vi "LiveSignal.vi"() -> ()   [LabVIEW 2022 SP3]
uses:
  <extravilib>/ChannelInstances/Tag-a[.](wfm(dbl)).lvlib
  ViolinSubs/Mic/Mic_Global.vi
  <extravilib>/ChannelInstances/Lossy Stream-a[.](wfm(dbl)).lvlib
  <vilib>/Analysis/NI_AALPro.lvlib
  ViolinSubs/PreferencesControl.ctl
panel:
  in  "Update Template":bool
  in  "max_scale":bool
  in  "last scale":bool
  in  "Load a Template":bool
  in  "autoscale":bool
  in  "Save as a Template":bool
  in  "device:":u16(ring) items=["BuerginBase Microphone", "485B39 200083408035100798118210422", "MacBook Pro Microphone", "Camo Microphone", "KM Audio Device", "Microsoft Teams Audio", "ZoomAudioDevice"]
  out "data":waveform(dbl)[](array[waveform])
  in  "Tab Control":T1(tab)
  in  "Magnitude Averages":u8(slide)=25 scale=1.0..50.0
  out "Hammer":waveform(dbl)(graph)
  out "Microphone":waveform(dbl)(graph)
  out "Mic Power Spectrum":waveform(dbl)(graph)
  out "Cal Hammer":waveform(dbl)[](graph)
  out "cal Mic":waveform(dbl)[](graph)
  out "Power Spectrum 2":waveform(dbl)(graph)
  in  "In->Out":bool
  in  "Out->In":bool
  out "Trig Mic":waveform(dbl)[](graph)
  out "Trig Hammer":waveform(dbl)[](graph)
  out "Triggered Spectrum":waveform(dbl)(graph)
  out "Real/Imag":cluster{dbl, "df":dbl, dbl[]}[](graph)
  out "Average FRF":cluster{dbl, "df":dbl, dbl[]}(graph)
  in  "Offset (msec)":dbl(slide) scale=0.0..10.0
  in  "Settings":T2={"Name of test"="", "Date"=timestamp(3691169924 s since 1904-01-01), "Location"="", "Template"="", "Soundcard"="485B39 200083408035100798118210422", "resolution"=32, "Sampling rate"=48000, "Ch1 Gain "=0.0, "Ch2 Gain"=0.0, "Sample time (s)"=0.3, "Pre-trigger (s)"=0.01, "Hammer Threshold"=0.01, "Positions"=12, "Taps/Position"=5, "Set Names"="", "Freq resolution"=1.0, "Hammer cutoff"=1.0, "Mic cutoff"=1.0, "Double bounce "=0.1, "Hammer Cal"=1000.0, "dB Offset"=0.0, "Accel Cal"=1000.0, "Vibrometer Cal"=1000.0, "Mic Cal"=1000.0, "Output"=2, "Voltage Cal"=1.0, "Vibrometer Port"="ASRL27::INSTR", "Range"=50, "High Pass"=2, "Bandwidth"=25, "X Range"=[], "Y Range"=[], "dB Spread"=40.0, "Trigger"=0, "Ch_1"=1, "Ch_2"=2, "flip?"=FALSE, "60Hz"=FALSE, "Time offset"=0.0, "Piezo Cal"=1.0, "Default Notes"="", "Tom"=FALSE} {"Ch_2" min=1 step=1; "Ch_1" min=1 max=100 step=1; "Trigger" items=["Hammer (force)", "Self-tap", "Spacebar"]; "Bandwidth" items=["1 kHz"=1, "5 kHz"=5, "10 kHz"=10, "25 kHz"=25, "50 kHz"=50, "100 kHz"=100]; "High Pass" items=["Off", "13 Hz", "104 Hz"]; "Range" items=["10 mm/s"=1, "20 mm/s"=2, "50 mm/s"=5, "100 mm/s"=10, "200 mm/s"=20, "500 mm/s"=50, "1 m/s"=100, "2 m/s"=200]; "Output" items=["Accelerometer", "Speed (from acceleration)", "Microphone", "Vibrometer", "Piezo"]; "Voltage Cal" format="%#_13g"; "Ch2 Gain" format="%#_13g"; "Ch1 Gain" format="%#_13g"; "Double bounce" min=0.0; "Mic cutoff" min=0.0 format="%#_4g"; "Hammer cutoff" min=0.0 format="%#_4g"; "Freq resolution" min=0.0; "Pre-trigger (s)" format="%#_13g"; "Date" format="%<%H:%M\n%d/%m/%y>T"; "resolution" items=["16 bit"=16, "24 bit"=24, "32 bit"=32]; "Sampling rate" items=["22050 samp/s"=22050, "44100 samp/s"=44100, "48000 samp/s"=48000]}
  # "For Mac mic - start running and then have both channels on 1"
  # "Raw values from the Soundcard"
  # "Calibrated Values"
  # "All values are calibrated, arrows sync x axes"
  # "Hz"
  # "dB"
  # "dB"
  # "sec"
  # "sec"
  # "mV/Pa"
  # "mV/m/s2"
  # "mV/mm/s"
  # "V/N"
  # "sec"
  # "sec"
  # "mV/N"
  # "%"
  # "%"
  # "sec"
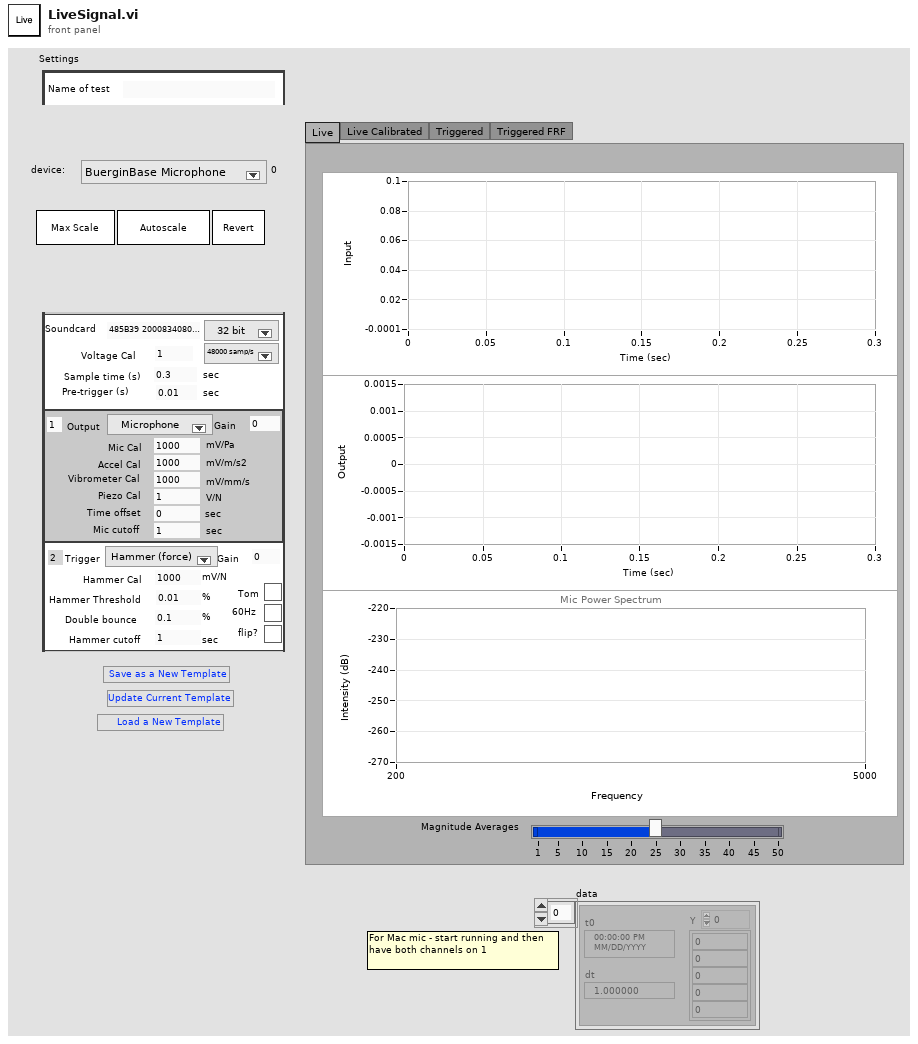
[diagram p1: front panel]
types:
  T1 = enum32{"Live", "Live Calibrated", "Triggered", "Triggered FRF"}
  T2 = typedef "PreferencesControl.ctl" = cluster{"Name of test":string, "Date":timestamp, "Location":string, "Template":string, "Soundcard":string, "resolution":u16, "Sampling rate":u16, "Ch1 Gain ":dbl, "Ch2 Gain":dbl, "Sample time (s)":dbl, "Pre-trigger (s)":dbl, "Hammer Threshold":dbl, "Positions":i16, "Taps/Position":i16, "Set Names":string, "Freq resolution":dbl, "Hammer cutoff":dbl, "Mic cutoff":dbl, "Double bounce ":dbl, "Hammer Cal":dbl, "dB Offset":dbl, "Accel Cal":dbl, "Vibrometer Cal":dbl, "Mic Cal":dbl, "Output":u16, "Voltage Cal":dbl, "Vibrometer Port":refnum<visa-resource-name>, "Range":u16, "High Pass":u16, "Bandwidth":u16, "X Range":cluster{"Minimum":dbl, "Maximum":dbl, "Increment":dbl, "Minor Increment":dbl, "Start":dbl}[], "Y Range":cluster{"Minimum":dbl, "Maximum":dbl, "Increment":dbl, "Minor Increment":dbl, "Start":dbl}[], "dB Spread":dbl, "Trigger":u16, "Ch_1":u8, "Ch_2":u8, "flip?":bool, "60Hz":bool, "Time offset":dbl, "Piezo Cal":dbl, "Default Notes":string, "Tom":bool}
  T3 = typedef "Tag-a[.](wfm(dbl)).lvlib/))Channel.ctl" = refnum<queue>
  T4 = typedef "Lossy Stream-a[.](wfm(dbl)).lvlib/)Channel.ctl" = refnum<queue>
  T5 = enum8{"Enabled", "Disabled", "Disabled and Grayed Out"}
  T6 = enum16{"Read", "Write", "Init", "remember", "retrieve"}
  T7 = typedef "LVRangeTypeDef.ctl" = cluster{"Minimum":dbl, "Maximum":dbl, "Increment":dbl, "Minor Increment":dbl, "Start":dbl}
  T8 = enum16{"Initialize", "Free run", "One Shot - waiting", "One Shot - triggered", "Wait", "Close"}
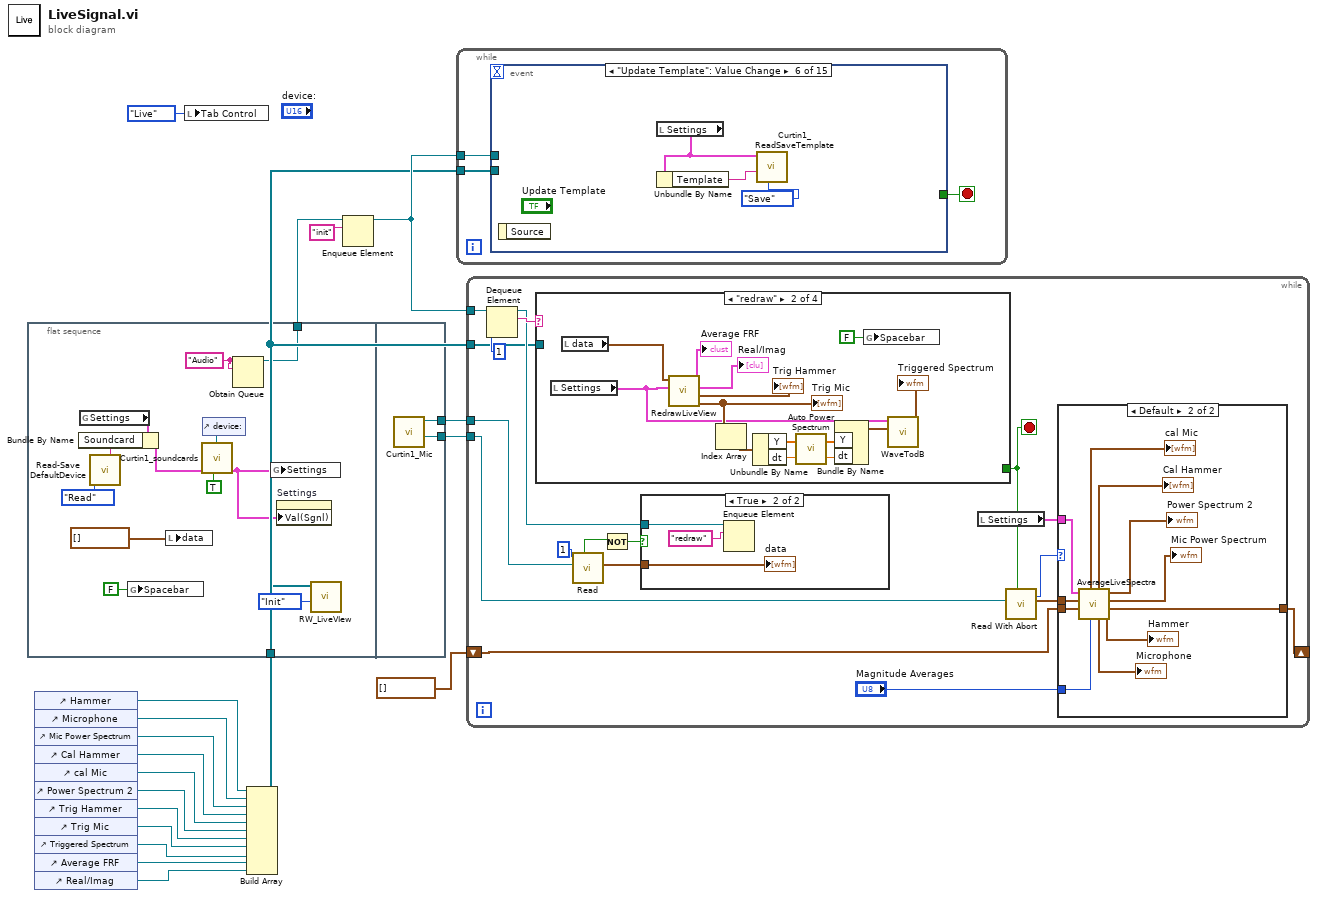
[diagram p0: block diagram]
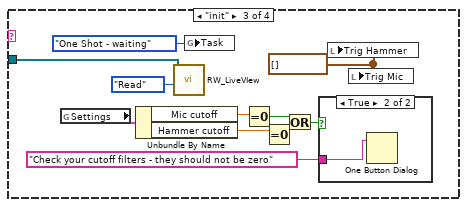
[diagram p5: hidden frame]
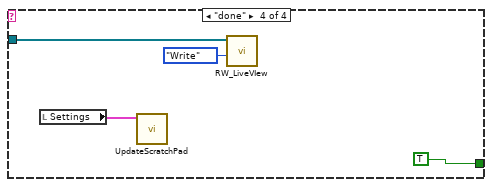
[diagram p7: hidden frame]
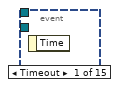
[diagram p8: hidden frame]
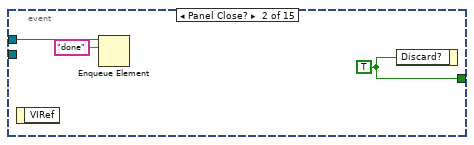
[diagram p9: hidden frame]
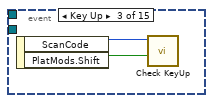
[diagram p10: hidden frame]
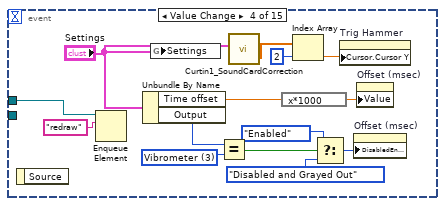
[diagram p11: hidden frame]
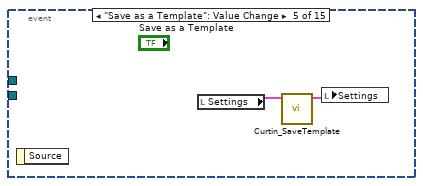
[diagram p12: hidden frame]
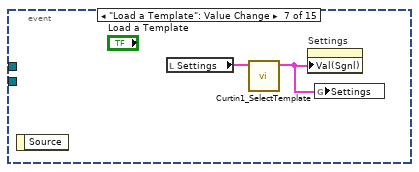
[diagram p13: hidden frame]
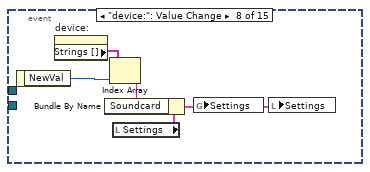
[diagram p14: hidden frame]
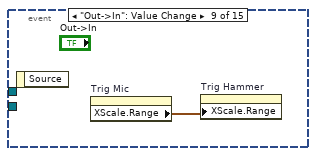
[diagram p15: hidden frame]
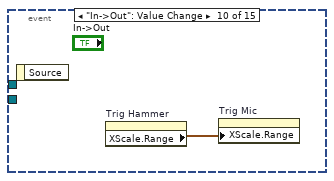
[diagram p16: hidden frame]
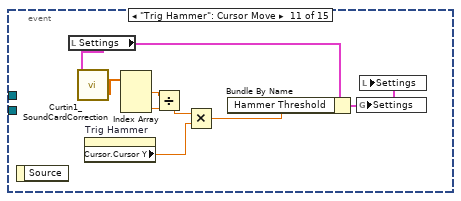
[diagram p17: hidden frame]
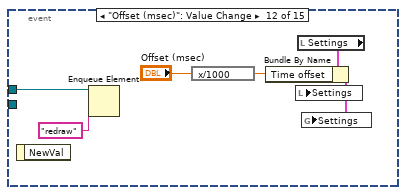
[diagram p18: hidden frame]
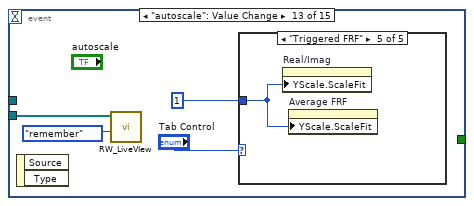
[diagram p19: hidden frame]
diagram:
  n1 = flat-sequence {
    tunnel: [w26] -> w15
    tunnel: w1 -> [w22]
    tunnel: [w34] -> w19
    tunnel: [w33] -> w18
    frame #0 {
      w27 = "Audio" ("name (unnamed)")
      n2 = global read "Mic_Global.vi" "Settings"() -> (w30:T2)
      n3 = call "Read-Save DefaultDevice.vi"("Task"=enum16{"Save", "Read"}."Read") -> ("Soundcard Out"=w29:string)  [unwired: 9 in, 1 out]
      n4 = Bundle By Name(cluster=w30, "Soundcard"=w29) -> (w25:T2)
      n5 = global write "Mic_Global.vi" "Spacebar"(FALSE ("Spacebar")) -> ()
      n6 = local write "data"(waveform(dbl)[] [] ("data")) -> ()
      n7 = control-ref of="device:"() -> (w32:refnum<vi>)
      n8 = call "Curtin1_soundcards.vi"("hush?"=TRUE, "Settings In"=w25, "device:"=w32) -> ("Settings Out"=w24:T2)  [unwired: 7 in, 1 out]
      n9 = Obtain Queue(name (unnamed)=w27, element data type=w27) -> (queue out=w26:refnum<queue>)  [unwired: 3 in, 2 out]
      n10 = global write "Mic_Global.vi" "Settings"(w24) -> ()
      n11 = property on="Settings" class="Clust (strict)"("Val(Sgnl)"=w24) -> ()  [unwired: 2 in, 2 out]
      n12 = call "RW_LiveVIew.vi"("Task"=enum16{"Read", "Write", "Init"}."Init", "Plots"=w22) -> ()  [unwired: 10 in]
    }
    frame #1 {
      n13 = call "Curtin1_Mic.vi"() -> ("latest data"=w33:T3, "Tap"=w34:T4)  [unwired: 10 in]
    }
  }
  n14 = control-ref of="Hammer"() -> (w13:refnum<vi>)
  n15 = control-ref of="Microphone"() -> (w12:refnum<vi>)
  n16 = control-ref of="Mic Power Spectrum"() -> (w11:refnum<vi>)
  n17 = control-ref of="Cal Hammer"() -> (w10:refnum<vi>)
  n18 = control-ref of="cal Mic"() -> (w9:refnum<vi>)
  n19 = control-ref of="Power Spectrum 2"() -> (w8:refnum<vi>)
  n20 = control-ref of="Trig Hammer"() -> (w7:refnum<vi>)
  n21 = control-ref of="Trig Mic"() -> (w6:refnum<vi>)
  n22 = control-ref of="Triggered Spectrum"() -> (w5:refnum<vi>)
  n23 = control-ref of="Average FRF"() -> (w4:refnum<vi>)
  n24 = control-ref of="Real/Imag"() -> (w3:refnum<vi>)
  n25 = local write "Tab Control"(T1."Live" ("Tab Control")) -> ()
  n26 = Build Array(w13, w12, w11, w10, w9, w8, w7, w6, w5, w4, w3) -> (w1:refnum<vi>[])
  n27 = Enqueue Element(queue=w15, element="init") -> (queue out=w16:refnum<queue>)  [unwired: 2 in, 2 out]
  n28 = while {
    tunnel: w16 -> [w37]
    tunnel: w1 -> [w35]
    stop <- w36 stop-if-true
    n29 = event shown="[5] \"Update Template\": Value Change" {
      selector: _ -> [_ _ _ _ _ _ _ _ _ _ _ _ _ _ _]
      dyn-events: _ -> [_ _ _ _ _ _ _ _ _ _ _ _ _ _ _]
      timeout: _ -> [_ _ _ _ _ _ _ _ _ _ _ _ _ _ _]
      tunnel: [_ w40 _ _ _ _ _ _ _ _ _ _ _ _ _] -> w36
      tunnel: w37 -> [_ w39 _ w55 _ _ _ _ _ _ _ w79 _ _ _]
      tunnel: w35 -> [_ _ _ _ _ _ _ _ _ _ _ _ w86 w93 _]
      event Timeout {
        n30 = event-data() -> ()  [unwired: 1 in, 1 out]
      }
      event Panel Close? {
        w40 = TRUE ("Discard?")
        n31 = event-data() -> ()  [unwired: 1 in, 1 out]
        n32 = Enqueue Element(queue=w39, element="done") -> ()  [unwired: 2 in, 3 out]
        n33 = event-data("Discard?"=w40) -> ()  [unwired: 1 in, 1 out]
      }
      event Key Up {
        n34 = event-data() -> ("ScanCode"=w42:i16, "PlatMods.Shift"=w41:bool)  [unwired: 1 in]
        n35 = call "Check KeyUp.vi"("Shift"=w41, "ScanCode"=w42) -> ()  [unwired: 9 in, 1 out]
      }
      event Value Change {
        w44 = u16 3 items=["Accelerometer", "Accel (speed)", "Microphone", "Vibrometer"] ("Output")
        n36 = event-data() -> ()  [unwired: 1 in, 1 out]
        n37 = Enqueue Element(queue=w55, element="redraw") -> ()  [unwired: 2 in, 3 out]
        n38 = Unbundle By Name("Settings") -> ("Time offset"=w54:dbl, "Output"=w45:u16)
        n39 = global write "Mic_Global.vi" "Settings"("Settings") -> ()
        n40 = Equal?(x=w45, y=w44) -> (x = y?=w46:bool)
        n41 = call "Curtin1_SoundCardCorrection.vi"("Settings"="Settings") -> ("Converted"=w51:dbl[])  [unwired: 5 in, 5 out]
        n42 = expression code="x*1000"(w54) -> (w53:dbl)
        n43 = Index Array(array=w51, index=2) -> (element=w49:dbl)
        n44 = Select(t=T5."Enabled" ("Disabled"), s=w46, f=T5."Disabled and Grayed Out" ("Disabled")) -> (s? t:f=w48:T5)
        n45 = property on="Trig Hammer" class="WFGraph (strict)"("Cursor.Cursor Y"=w49) -> ()  [unwired: 2 in, 2 out]
        n46 = property on="Offset (msec)" class="Slide (strict)"("DisabledEnum"=w48) -> ()  [unwired: 2 in, 2 out]
        n47 = property on="Offset (msec)" class="Slide (strict)"("Value"=w53) -> ()  [unwired: 2 in, 2 out]
      }
      event "Save as a Template": Value Change {
        n48 = event-data() -> ()  [unwired: 1 in, 1 out]
        n49 = local read "Settings"() -> (w58:T2)
        n50 = call "Curtin_SaveTemplate.vi"("Settings in"=w58) -> ("Settings out"=w57:T2)  [unwired: 8 in, 2 out]
        n51 = local write "Settings"(w57) -> ()
      }
      event "Update Template": Value Change {
        n52 = event-data() -> ()  [unwired: 1 in, 1 out]
        n53 = local read "Settings"() -> (w59:T2)
        n54 = Unbundle By Name(w59) -> ("Template"=w60:string)
        n55 = call "Curtin1_ReadSaveTemplate.vi"("Task"=enum16{"Save", "Read", "List"}."Save", "Template"=w60, "Settings"=w59) -> ()  [unwired: 5 in, 4 out]
      }
      event "Load a Template": Value Change {
        n56 = event-data() -> ()  [unwired: 1 in, 1 out]
        n57 = local read "Settings"() -> (w63:T2)
        n58 = call "Curtin1_SelectTemplate.vi"("Settings in"=w63) -> ("Settings out"=w62:T2)  [unwired: 9 in, 1 out]
        n59 = property on="Settings" class="Clust (strict)"("Val(Sgnl)"=w62) -> ()  [unwired: 2 in, 2 out]
        n60 = global write "Mic_Global.vi" "Settings"(w62) -> ()
      }
      event "device:": Value Change {
        n61 = event-data() -> ("NewVal"=w67:u16)  [unwired: 1 in]
        n62 = property on="device:" class="Ring (strict)"() -> ("Strings []"=w68:string[])  [unwired: 2 in, 2 out]
        n63 = Index Array(array=w68, index=w67) -> (element=w65:string)
        n64 = local read "Settings"() -> (w66:T2)
        n65 = Bundle By Name(cluster=w66, "Soundcard"=w65) -> (w64:T2)
        n66 = global write "Mic_Global.vi" "Settings"(w64) -> ()
        n67 = local write "Settings"(w64) -> ()
      }
      event "Out->In": Value Change {
        n68 = event-data() -> ()  [unwired: 1 in, 1 out]
        n69 = property on="Trig Mic" class="WFGraph (strict)"() -> ("XScale.Range"=w69:T7)  [unwired: 2 in, 2 out]
        n70 = property on="Trig Hammer" class="WFGraph (strict)"("XScale.Range"=w69) -> ()  [unwired: 2 in, 2 out]
      }
      event "In->Out": Value Change {
        n71 = event-data() -> ()  [unwired: 1 in, 1 out]
        n72 = property on="Trig Hammer" class="WFGraph (strict)"() -> ("XScale.Range"=w70:T7)  [unwired: 2 in, 2 out]
        n73 = property on="Trig Mic" class="WFGraph (strict)"("XScale.Range"=w70) -> ()  [unwired: 2 in, 2 out]
      }
      event "Trig Hammer": Cursor Move {
        n74 = event-data() -> ()  [unwired: 1 in, 1 out]
        n75 = local read "Settings"() -> (w71:T2)
        n76 = call "Curtin1_SoundCardCorrection.vi"("Settings"=w71) -> ("Converted"=w77:dbl[])  [unwired: 5 in, 5 out]
        n77 = property on="Trig Hammer" class="WFGraph (strict)"() -> ("Cursor.Cursor Y"=w73:dbl)  [unwired: 2 in, 2 out]
        n78 = Index Array(array=w77) -> (element #1=w76:dbl, element #3=w75:dbl)  [unwired: 3 in, 1 out]
        n79 = Divide(x=w76, y=w75) -> (x/y=w74:dbl)
        n80 = Multiply(x=w74, y=w73) -> (x*y=w72:dbl)
        n81 = Bundle By Name(cluster=w71, "Hammer Threshold"=w72) -> (w78:T2)
        n82 = global write "Mic_Global.vi" "Settings"(w78) -> ()
        n83 = local write "Settings"(w78) -> ()
      }
      event "Offset (msec)": Value Change {
        n84 = event-data() -> ()  [unwired: 1 in, 1 out]
        n85 = Enqueue Element(queue=w79, element="redraw") -> ()  [unwired: 2 in, 3 out]
        n86 = expression code="x/1000"("Offset (msec)") -> (w81:dbl)
        n87 = local read "Settings"() -> (w84:T2)
        n88 = Bundle By Name(cluster=w84, "Time offset"=w81) -> (w83:T2)
        n89 = local write "Settings"(w83) -> ()
        n90 = global write "Mic_Global.vi" "Settings"(w83) -> ()
      }
      event "autoscale": Value Change {
        n91 = event-data() -> ()  [unwired: 1 in, 2 out]
        n92 = call "RW_LiveVIew.vi"("Task"=T6."remember", "Plots"=w86) -> ()  [unwired: 10 in]
        n93 = case shown="\"Triggered FRF\"" "Tab Control" {
          tunnel: u8 1 ("Y Scale.Scale Fit") -> [_ w89 w90 w91 w92]
          frame Default {
          }
          frame "Live" {
            n94 = property on="Hammer" class="WFGraph (strict)"("YScale.ScaleFit"=w89) -> ()  [unwired: 2 in, 2 out]
            n95 = property on="Mic Power Spectrum" class="WFGraph (strict)"("YScale.ScaleFit"=w89) -> ()  [unwired: 2 in, 2 out]
            n96 = property on="Microphone" class="WFGraph (strict)"("YScale.ScaleFit"=w89) -> ()  [unwired: 2 in, 2 out]
          }
          frame "Live Calibrated" {
            n97 = property on="Cal Hammer" class="WFGraph (strict)"("YScale.ScaleFit"=w90) -> ()  [unwired: 2 in, 2 out]
            n98 = property on="cal Mic" class="WFGraph (strict)"("YScale.ScaleFit"=w90) -> ()  [unwired: 2 in, 2 out]
          }
          frame "Triggered" {
            n99 = property on="Trig Hammer" class="WFGraph (strict)"("YScale.ScaleFit"=w91) -> ()  [unwired: 2 in, 2 out]
            n100 = property on="Trig Mic" class="WFGraph (strict)"("YScale.ScaleFit"=w91) -> ()  [unwired: 2 in, 2 out]
            n101 = property on="Triggered Spectrum" class="WFGraph (strict)"("YScale.ScaleFit"=w91) -> ()  [unwired: 2 in, 2 out]
          }
          frame "Triggered FRF" {
            n102 = property on="Real/Imag" class="WFGraph (strict)"("YScale.ScaleFit"=w92) -> ()  [unwired: 2 in, 2 out]
            n103 = property on="Average FRF" class="WFGraph (strict)"("YScale.ScaleFit"=w92) -> ()  [unwired: 2 in, 2 out]
          }
        }
      }
      event "last scale": Value Change {
        n104 = event-data() -> ()  [unwired: 1 in, 2 out]
        n105 = call "RW_LiveVIew.vi"("Task"=T6."retrieve", "Plots"=w93) -> ()  [unwired: 10 in]
      }
      event "max_scale": Value Change {
        n106 = event-data() -> ()  [unwired: 1 in, 2 out]
        n107 = property on="Microphone" class="WFGraph (strict)"("YScale.Minimum"=-1.0 ("Y Scale.Range:Maximum"), "YScale.Maximum"=1.0 ("Y Scale.Range:Maximum")) -> ()  [unwired: 2 in, 2 out]
        n108 = property on="Hammer" class="WFGraph (strict)"("YScale.Minimum"=-1.0 ("Y Scale.Range:Maximum"), "YScale.Maximum"=1.0 ("Y Scale.Range:Maximum")) -> ()  [unwired: 2 in, 2 out]
      }
    }
  }
  n109 = while {
    tunnel: w16 -> [w116]
    tunnel: w19 -> [w108]
    tunnel: w18 -> [w113]
    tunnel: w1 -> [w104]
    shift-right: [w101] -> _
    shift-left: waveform(dbl)[] [] -> [w103]
    stop <- w112 stop-if-true
    n110 = Dequeue Element(queue=w116, timeout in ms (-1)=1) -> (queue out=w106:refnum<queue>, element=w115:string)  [unwired: 1 in, 2 out]
    n111 = case shown="\"redraw\"" w115 {
      tunnel: [_ _ _ TRUE ("Discard?")] -> w112
      tunnel: w104 -> [_ _ w146 w158]
      frame Default {
      }
      frame "redraw" {
        n112 = local read "Settings"() -> (w133:T2)
        n113 = local read "data"() -> (w145:waveform(dbl)[])
        n114 = call "RedrawLiveView.vi"("Settings"=w133, "data"=w145) -> ("Trig Mic"=w137:waveform(dbl)[], "Trig Hammer"=→"Trig Hammer":waveform(dbl)[], "Real/Imag"=→"Real/Imag":cluster{dbl, "df":dbl, dbl[]}[], "Average FRF"=→"Average FRF":cluster{dbl, "df":dbl, dbl[]})  [unwired: 6 in]
        "Trig Mic" <- w137
        n115 = Index Array(array=w137) -> (element=w136:waveform(dbl))  [unwired: 1 in]
        n116 = Unbundle By Name(w136) -> ("Y"=w141:dbl[], "dt"=w140:dbl)
        n117 = call <vilib>:"Auto Power Spectrum.vi"("dt"=w140, "Signal (V)"=w141) -> ("df"=w138:dbl, "Power Spectrum (V^2 rms)"=w139:dbl[])
        n118 = Bundle By Name("Y"=w139, "dt"=w138) -> (w134:waveform(dbl))  [unwired: 1 in]
        n119 = global write "Mic_Global.vi" "Spacebar"(FALSE ("Spacebar")) -> ()
        n120 = call "WaveTodB.vi"("spectrum in"=w134, "Settings"=w133) -> ("spectrum out"=→"Triggered Spectrum":waveform(dbl))  [unwired: 9 in]
      }
      frame "init" {
        w155 = waveform(dbl)[] [] ("Hammer 2")
        n121 = global read "Mic_Global.vi" "Settings"() -> (w154:T2)
        n122 = Unbundle By Name(w154) -> ("Mic cutoff"=w153:dbl, "Hammer cutoff"=w152:dbl)
        n123 = call "RW_LiveVIew.vi"("Task"=enum16{"Read", "Write", "Init"}."Read", "Plots"=w146) -> ()  [unwired: 10 in]
        n124 = global write "Mic_Global.vi" "Task"(T8."One Shot - waiting" ("Task")) -> ()
        n125 = Equal To 0?(x=w153) -> (x = 0?=w151:bool)
        n126 = Equal To 0?(x=w152) -> (x = 0?=w150:bool)
        n127 = Or(x=w151, y=w150) -> (x .or. y?=w148:bool)
        n128 = case shown="True" w148 {
          tunnel: "Check your cutoff filters - they should not be zero" ("element") -> [_ w157]
          frame False {
          }
          frame True {
            n129 = One Button Dialog(message=w157) -> ()  [unwired: 1 in, 1 out]
          }
        }
        n130 = local write "Trig Hammer"(w155) -> ()
        n131 = local write "Trig Mic"(w155) -> ()
      }
      frame "done" {
        n132 = local read "Settings"() -> (w160:T2)
        n133 = call "UpdateScratchPad.vi"("Settings"=w160) -> ()  [unwired: 9 in, 2 out]
        n134 = call "RW_LiveVIew.vi"("Task"=enum16{"Read", "Write", "Init"}."Write", "Plots"=w158) -> ()  [unwired: 10 in]
      }
    }
    n135 = call <extravilib>:"Read.vi"("channel"=w108, "timeout in ms (-1)"=1) -> ("element"=w111:waveform(dbl)[], "timed out?"=w110:bool)  [unwired: 4 in, 4 out]
    n136 = Not(x=w110) -> (.not. x?=w109:bool)
    n137 = case shown="True" w109 {
      tunnel: w111 -> [_ w131]
      tunnel: w106 -> [_ w129]
      frame False {
      }
      frame True {
        n138 = Enqueue Element(queue=w129, element="redraw") -> ()  [unwired: 2 in, 3 out]
        "data" <- w131
      }
    }
    n139 = local read "Settings"() -> (w105:T2)
    n140 = call <extravilib>:"Read With Abort.vi"("abort"=w112, "channel"=w113) -> ("element"=w100:waveform(dbl)[], "missed"=w99:i32)  [unwired: 7 in, 1 out]
    n141 = case shown="Default" w99 {
      tunnel: w105 -> [_ w128]
      tunnel: w100 -> [_ w127]
      tunnel: w103 -> [w117 w126]
      tunnel: "Magnitude Averages" -> [_ w125]
      tunnel: [w117 w118] -> w101
      frame -1 {
      }
      frame Default {
        n142 = call "AverageLiveSpectra.vi"("Magnitude Averages"=w125, "old reading"=w126, "new reading"=w127, "Settings"=w128) -> ("Hammer"=→"Hammer":waveform(dbl), "FIFO out"=w118:waveform(dbl)[], "average spectrum"=→"Mic Power Spectrum":waveform(dbl), "Power Spectrum"=→"Power Spectrum 2":waveform(dbl), "Microphone"=→"Microphone":waveform(dbl), "Cal Hammer"=→"Cal Hammer":waveform(dbl)[], "cal Mic"=→"cal Mic":waveform(dbl)[])  [unwired: 1 in]
      }
    }
  }
